vi "Graphing.vi"() -> ()   [LabVIEW 2018]
panel:
  out "Waveform Chart 2":cluster{dbl, "number: 0 to 1":dbl}(graph)
  out "R vs Vg : TimeGraph 2":cluster{dbl, "Current":sgl}[](graph)
  out "Waveform Chart":dbl(graph)
  out "R vs Vg : TimeGraph":cluster{dbl, "Current":sgl}[](graph)
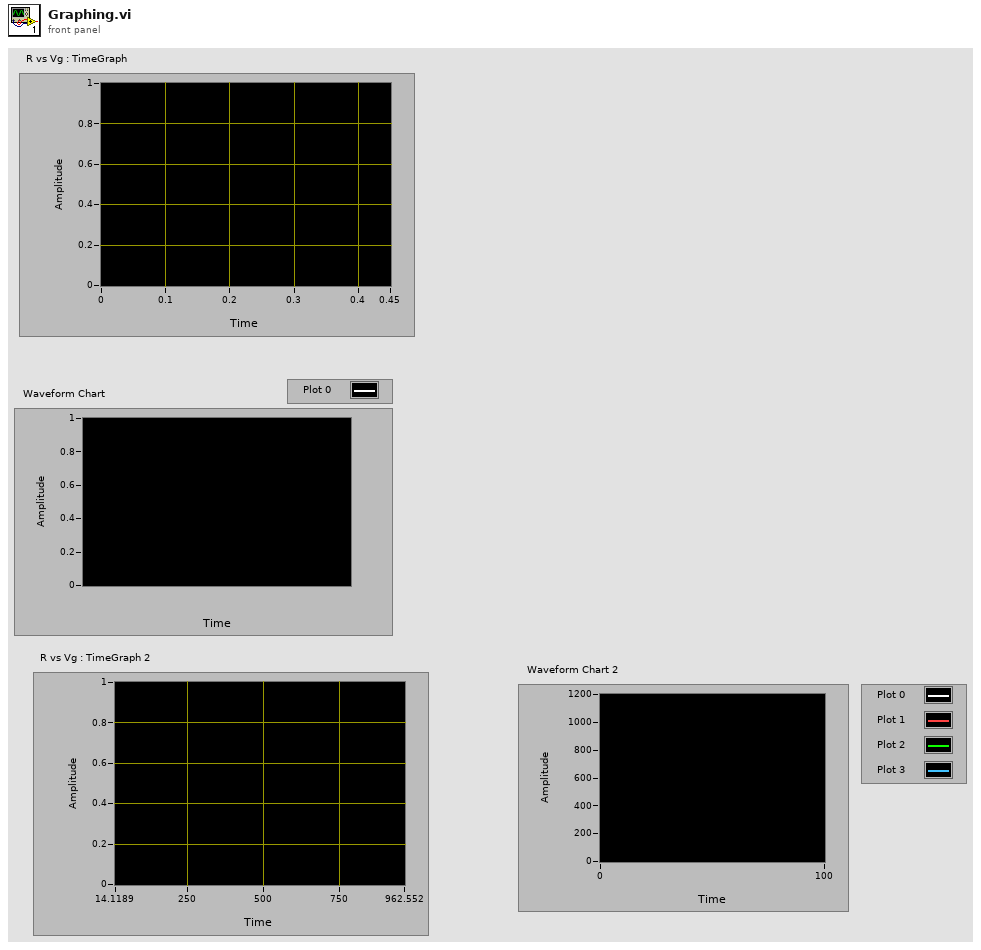
[diagram p1: front panel]
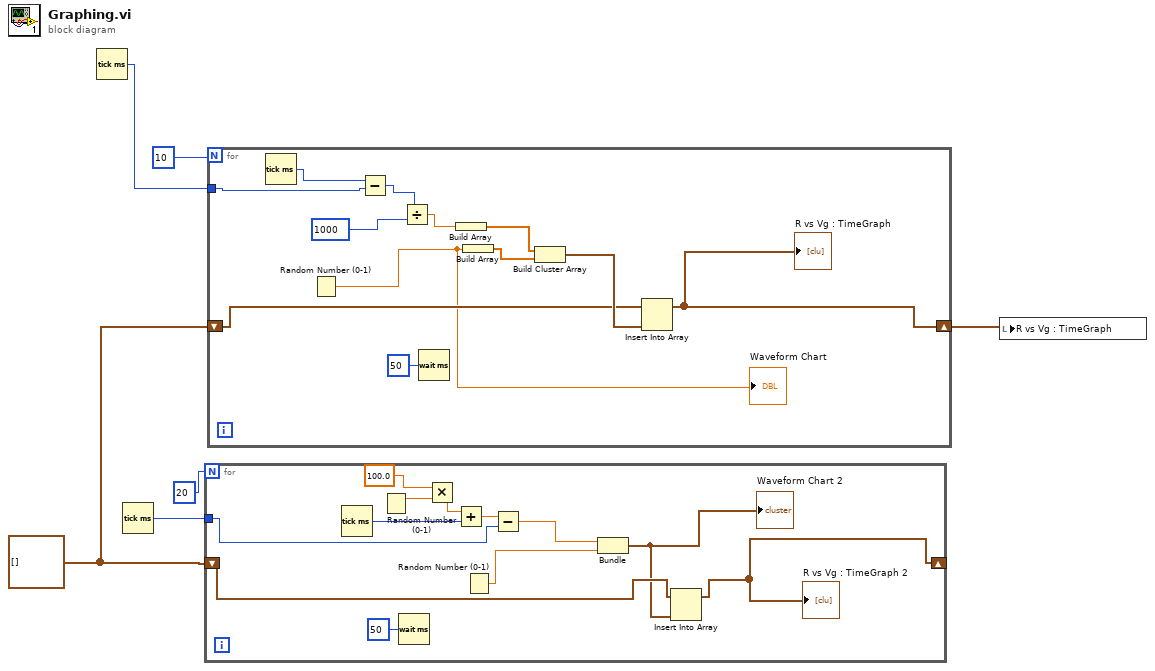
[diagram p0: block diagram]
diagram:
  w3 = cluster{dbl, "Current":sgl}[] [] ("History Data")
  n1 = Tick Count (ms)() -> (millisecond timer value=w4:u32)
  n2 = Tick Count (ms)() -> (millisecond timer value=w1:u32)
  n3 = for {
    N: 20 -> [_]
    shift-right: [w10] -> _
    shift-left: w3 -> [w11]
    tunnel: w1 -> [w12]
    n4 = Tick Count (ms)() -> (millisecond timer value=w13:u32)
    n5 = Random Number (0-1)() -> (number: 0 to 1=w17:dbl)
    n6 = Wait (ms)(milliseconds to wait=u32 50) -> ()  [unwired: 1 out]
    n7 = Multiply(x=100.0, y=w17) -> (x*y=w14:dbl)
    n8 = Add(x=w14, y=w13) -> (x+y=w15:dbl)
    n9 = Random Number (0-1)() -> (number: 0 to 1=w9:dbl)
    n10 = Subtract(x=w15, y=w12) -> (x-y=w8:dbl)
    n11 = Bundle(w8, "number: 0 to 1"=w9) -> (w7:cluster{dbl, "number: 0 to 1":dbl})  [unwired: 1 in]
    "Waveform Chart 2" <- w7
    n12 = Insert Into Array(array=w11, new element=w7) -> (w10:cluster{dbl, "Current":sgl}[])  [unwired: 1 in]
    "R vs Vg : TimeGraph 2" <- w10
  }
  n13 = for {
    N: 10 -> [_]
    tunnel: w4 -> [w26]
    shift-right: [w23] -> w6
    shift-left: w3 -> [w24]
    n14 = Tick Count (ms)() -> (millisecond timer value=w27:u32)
    n15 = Random Number (0-1)() -> (number: 0 to 1=w19:dbl)
    "Waveform Chart" <- w19
    n16 = Subtract(x=w27, y=w26) -> (x-y=w21:u32)
    n17 = Divide(x=w21, y=u32 1000) -> (x/y=w20:dbl)
    n18 = Wait (ms)(milliseconds to wait=u32 50) -> ()  [unwired: 1 out]
    n19 = Build Array(w20) -> (w30:dbl[])
    n20 = Build Array(w19) -> (w29:dbl[])
    n21 = Build Cluster Array(w30, w29) -> (w25:cluster{dbl, "number: 0 to 1":dbl}[])
    n22 = Insert Into Array(array=w24, new element=w25) -> (w23:cluster{dbl, "Current":sgl}[])  [unwired: 1 in]
    "R vs Vg : TimeGraph" <- w23
  }
  n23 = local write "R vs Vg : TimeGraph"(w6) -> ()
